vi "CallFormulaExpressVI.vi"(9 "X5":dbl, 10 "X3":dbl, 11 "X1":dbl) -> (0 "error out":errorcluster, 3 "Result":i32)   [LabVIEW 2012]
uses:
  <vilib>/express/express arith-compare/Formula/XNode/ExpressFormulaBlockNode.xnode
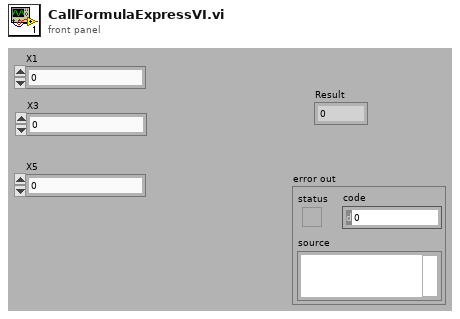
[diagram p1: front panel]
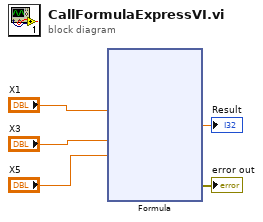
[diagram p0: block diagram]
diagram:
  n1 = xnode "Formula"("X1"="X1", "X3"="X3", "X5"="X5") -> ("Result"=→"Result":dbl, "error out"=→"error out":errorcluster)  [unwired: 1 in]
